vi "SIM Registry LookupByIdx.vi"(10 "Block Idx":i32=-1, 11 "Registry In":T1) -> (0 "Output Width":i32, 1 "Input Width":i32, 2 "Block Idx Out":i32, 3 "Registry Out":T1, 4 "Num Disc States":i32, 5 "Num Cont States":i32, 6 "Disc State Idx":i32, 7 "Cont State Idx":i32, 8 "Discrete ID":i32)   [LabVIEW 2020]
uses:
  <vilib>/Simulation/Implementation/Shared/SIM Registry.llb/SIM Simulation Registry.ctl
  <vilib>/Simulation/Implementation/Shared/SIM Registry.llb/SIM Registry Node Header.ctl
  <vilib>/Simulation/Implementation/Shared/SIM Registry.llb/SIM Registry Node Record.ctl
  <vilib>/Simulation/Implementation/Shared/SIM trigger type.ctl
  <vilib>/Simulation/Implementation/Shared/SIM solver state data.ctl
  <vilib>/Simulation/Implementation/Shared/SIM limit type.ctl
  <vilib>/Simulation/Implementation/Shared/SIM discrete data.ctl
  <vilib>/Simulation/Implementation/Shared/SIM Discrete state data.ctl
  <vilib>/Simulation/Implementation/Shared/SIM Registry.llb/SIM Simulation Registry Error.ctl
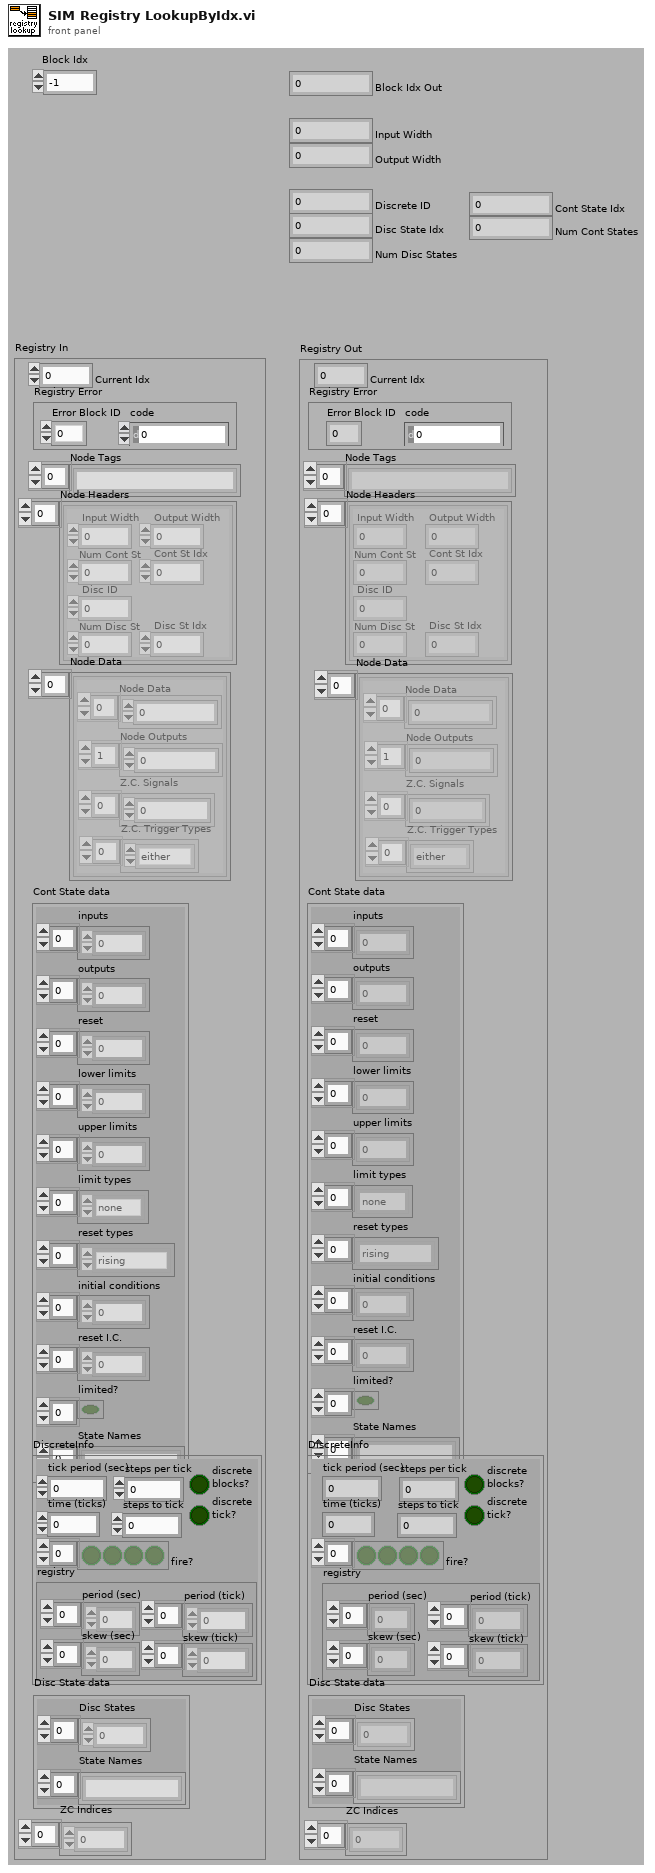
[diagram p1: front panel]
types:
  T1 = typedef "SIM Simulation Registry.ctl" = cluster{"Current Idx":i32, "Node Tags":string[], "Node Headers":T2[], "Node Data":T3[], "Cont State data":T5, "DiscreteInfo":T7, "Disc State data":T8, "Registry Error":T9, "ZC Indices":i32[]}
  T2 = typedef "SIM Registry Node Header.ctl" = cluster{"Input Width":i32, "Disc ID":i32, "Num Cont St":i32, "Cont St Idx":i32, "Num Disc St":i32, "Disc St Idx":i32, "Output Width":i32}
  T3 = typedef "SIM Registry Node Record.ctl" = cluster{"Node Data":dbl[], "Node Outputs":dbl[], "Z.C. Signals":dbl[], "Z.C. Trigger Types":T4[]}
  T4 = typedef "SIM trigger type.ctl" = enum16{"rising", "falling", "either", "none"}
  T5 = typedef "SIM solver state data.ctl" = cluster{"inputs":dbl[], "outputs":dbl[], "reset":dbl[], "lower limits":dbl[], "upper limits":dbl[], "limit types":T6[], "reset types":T4[], "initial conditions":dbl[], "reset I.C.":dbl[], "limited?":bool[], "State Names":string[]}
  T6 = typedef "SIM limit type.ctl" = enum16{"upper", "lower", "both", "none"}
  T7 = typedef "SIM discrete data.ctl" = cluster{"tick period (sec)":dbl, "time (ticks)":i32, "fire?":bool[], "registry":cluster{"period (sec)":dbl[], "skew (sec)":dbl[], "period (tick)":i32[], "skew (tick)":i32[]}, "discrete \nblocks?":bool, "steps per tick":dbl, "steps to tick":dbl, "discrete \ntick?":bool}
  T8 = typedef "SIM Discrete state data.ctl" = cluster{"Disc States":dbl[], "State Names":string[]}
  T9 = typedef "SIM Simulation Registry Error.ctl" = cluster{"Error Block ID":i32, "code":i32}
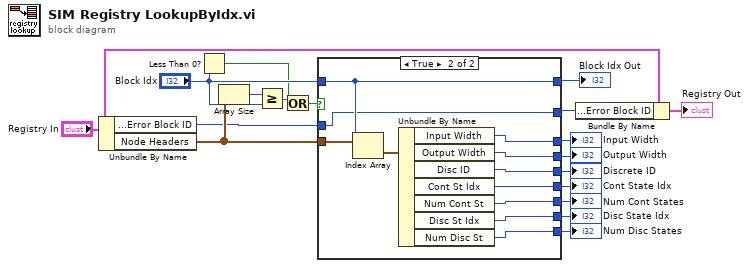
[diagram p0: block diagram]
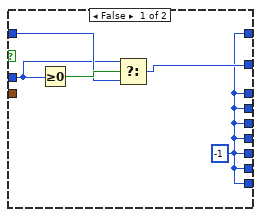
[diagram p2: hidden frame]
diagram:
  n1 = Unbundle By Name("Registry In") -> ("Registry Error.Error Block ID"=w7:i32, "Node Headers"=w15:T2[])
  n2 = Less Than 0?(x="Block Idx") -> (x < 0?=w11:bool)
  n3 = Array Size(array=w15) -> (size(s)=w14:i32)
  n4 = Greater Or Equal?(x=w14, y="Block Idx") -> (x >= y?=w12:bool)
  n5 = Or(x=w12, y=w11) -> (x .or. y?=w10:bool)
  n6 = case shown="True" w10 {
    tunnel: [w19 w30] -> w18
    tunnel: [w19 w32] -> w17
    tunnel: w15 -> [_ w34]
    tunnel: "Block Idx" -> [w21 w30]
    tunnel: [w19 w31] -> w16
    tunnel: w7 -> [w20 w29]
    tunnel: [w22 w29] -> w6
    tunnel: [w19 w28] -> w5
    tunnel: [w19 w27] -> w4
    tunnel: [w19 w26] -> w3
    tunnel: [w19 w25] -> w2
    tunnel: [w19 w24] -> w1
    frame False {
      w19 = -1 ("index of element")
      n7 = Greater Or Equal To 0?(x=w20) -> (x >= 0?=w23:bool)
      n8 = Select(t=w20, s=w23, f=w21) -> (s? t:f=w22:i32)
    }
    frame True {
      n9 = Index Array(array=w34, index=w30) -> (element=w33:T2)
      n10 = Unbundle By Name(w33) -> ("Input Width"=w32:i32, "Output Width"=w24:i32, "Disc ID"=w31:i32, "Cont St Idx"=w28:i32, "Num Cont St"=w27:i32, "Disc St Idx"=w26:i32, "Num Disc St"=w25:i32)
    }
  }
  "Block Idx Out" <- w18
  "Input Width" <- w17
  "Discrete ID" <- w16
  "Cont State Idx" <- w5
  "Num Cont States" <- w4
  "Disc State Idx" <- w3
  "Num Disc States" <- w2
  "Output Width" <- w1
  n11 = Bundle By Name(cluster="Registry In", "Registry Error.Error Block ID"=w6) -> (→"Registry Out":T1)
